vi "TempControlME.vi"(0 "Furnace Spoint":dbl, 5 "Stoic Temp":dbl, 7 "Target Temp":dbl, 9 "Previous Setpoint":dbl format="%#_13g", 11 "User Spoint":dbl, 12 "Countdown":i32) -> (4 "Furnace Setpoint":dbl format="%#_13g", 6 "Limit Exceeded":bool, 10 "User Setpoint":dbl format="%#_13g", 14 "Countdown":i32)   [LabVIEW 2014]
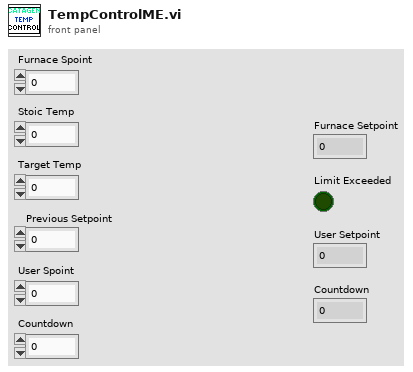
[diagram p1: front panel]
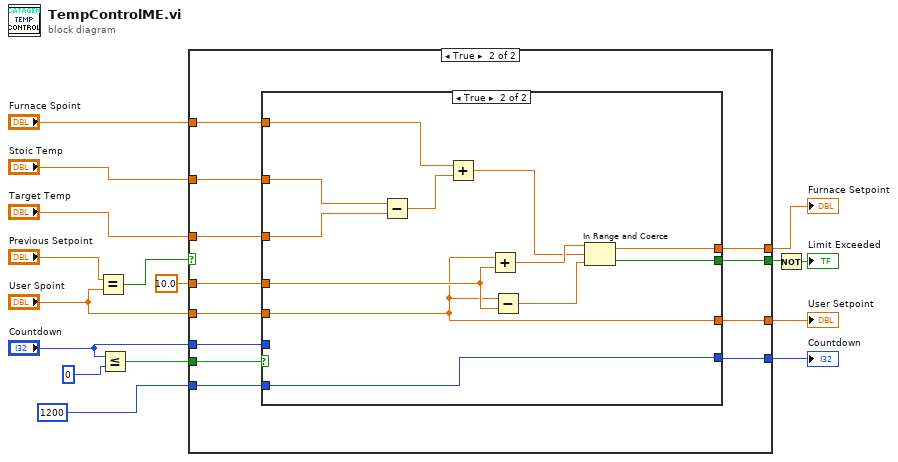
[diagram p0: block diagram]
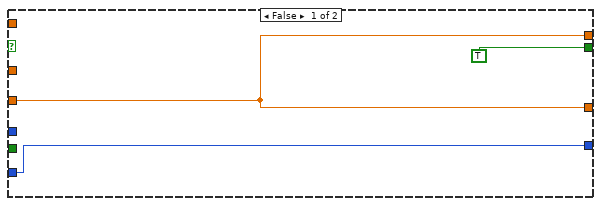
[diagram p2: hidden frame]
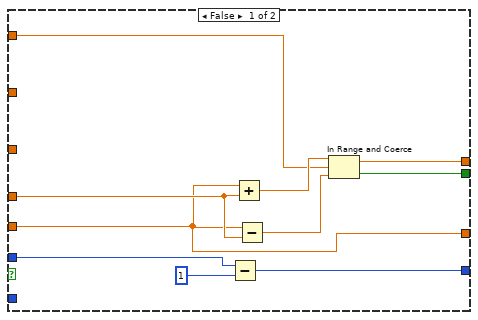
[diagram p3: hidden frame]
diagram:
  n1 = Equal?(x="Previous Setpoint", y="User Spoint") -> (x = y?=w1:bool)
  n2 = Less Or Equal?(x="Countdown", y=0) -> (x <= y?=w15:bool)
  n3 = case shown="True" w1 {
    tunnel: w15 -> [_ w31]
    tunnel: "Countdown" -> [_ w30]
    tunnel: [w18 w29] -> w13
    tunnel: 1200 ("Settling Time") -> [w18 w28]
    tunnel: "Stoic Temp" -> [_ w27]
    tunnel: "Target Temp" -> [_ w26]
    tunnel: "User Spoint" -> [w19 w25]
    tunnel: "Furnace Spoint" -> [_ w24]
    tunnel: [TRUE w23] -> w8
    tunnel: [w19 w22] -> w6
    tunnel: 10.0 -> [_ w21]
    tunnel: [w19 w20] -> w4
    frame False {
    }
    frame True {
      n4 = case shown="True" w31 {
        tunnel: w30 -> [w40 _]
        tunnel: [w39 w53] -> w29
        tunnel: w28 -> [_ w53]
        tunnel: w27 -> [_ w52]
        tunnel: w26 -> [_ w51]
        tunnel: w25 -> [w32 w42]
        tunnel: w24 -> [w36 w46]
        tunnel: [w34 w48] -> w22
        tunnel: [w35 w47] -> w23
        tunnel: w21 -> [w33 w43]
        tunnel: [w32 w42] -> w20
        frame False {
          n5 = Subtract(x=w40, y=1) -> (x-y=w39:i32)
          n6 = Add(x=w32, y=w33) -> (x+y=w38:dbl)
          n7 = Subtract(x=w32, y=w33) -> (x-y=w37:dbl)
          n8 = In Range and Coerce(upper limit=w38, x=w36, lower limit=w37) -> (coerced(x)=w34:dbl, In Range?=w35:bool)
        }
        frame True {
          n9 = Subtract(x=w52, y=w51) -> (x-y=w45:dbl)
          n10 = Add(x=w46, y=w45) -> (x+y=w44:dbl)
          n11 = Add(x=w42, y=w43) -> (x+y=w50:dbl)
          n12 = Subtract(x=w42, y=w43) -> (x-y=w49:dbl)
          n13 = In Range and Coerce(upper limit=w50, x=w44, lower limit=w49) -> (coerced(x)=w48:dbl, In Range?=w47:bool)
        }
      }
    }
  }
  "Countdown" <- w13
  "Furnace Setpoint" <- w6
  "User Setpoint" <- w4
  n14 = Not(x=w8) -> (.not. x?=→"Limit Exceeded":bool)
